vi "任意时刻多点闹钟.vi"(8 "Error In":errorcluster caption="错误输入", 10 "偏移量（秒）":dbl[](array[numeric]), 11 "定闹时刻":timestamp[](array[timestamp])) -> (0 "Error Out":errorcluster caption="错误输出", 2 "离定闹时间还有（秒）":dbl[](array[numeric]))   [LabVIEW 2012]
panel:
  out "时间到？":bool[](array[boolean])
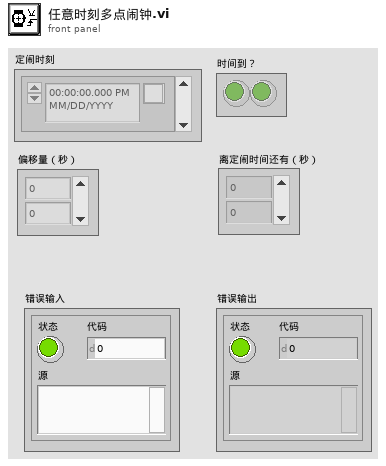
[diagram p1: front panel]
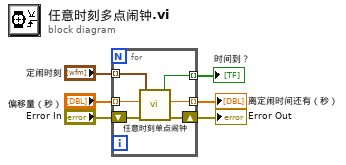
[diagram p0: block diagram]
diagram:
  n1 = for {
    tunnel: "定闹时刻" -> [w12] mode=indexing
    tunnel: "偏移量（秒）" -> [w11] mode=indexing
    shift-right: [w7] -> w3
    shift-left: "Error In" -> [w8]
    tunnel: [w10] -> w2 mode=indexing
    tunnel: [w9] -> w1 mode=indexing
    n2 = call "任意时刻单点闹钟.vi"("Error In"=w8, "偏移量（秒）"=w11, "定闹时刻"=w12) -> ("Error Out"=w7:errorcluster, "离定闹时间还有（秒）"=w9:dbl, "时间到"=w10:bool)  [unwired: 6 in]
  }
  "离定闹时间还有（秒）" <- w1
  "Error Out" <- w3
  "时间到？" <- w2
